vi "closeLog.vi"(8 "error in (no error)":errorcluster, 11 "Logger in":refnum<class "Log.lvclass">) -> (0 "error out":errorcluster, 3 "Logger out":refnum<class "Log.lvclass">)   [LabVIEW 2013, in "Log.lvclass"]
uses:
  Log.lvclass
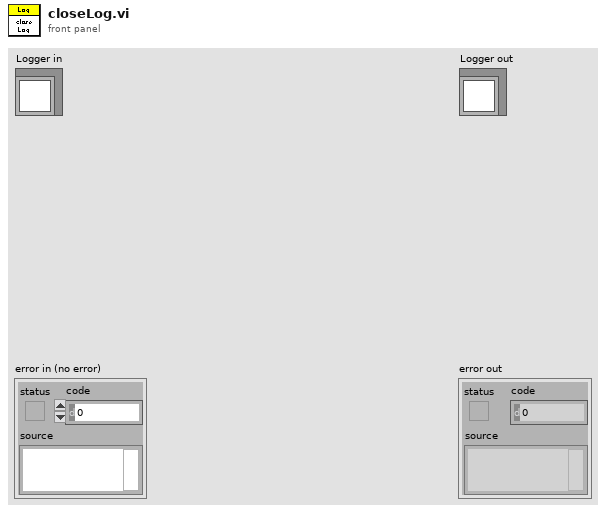
[diagram p1: front panel]
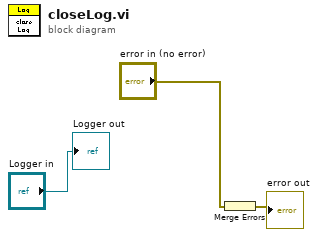
[diagram p0: block diagram]
diagram:
  n1 = Merge Errors("error in (no error)") -> (→"error out":errorcluster)
  "Logger out" <- "Logger in"
